vi "Actor Core.vi"(8 "Error In":errorcluster, 11 "CS++RTWatchdogActor in":refnum<class "CS++RTWatchdogActor.lvclass">) -> (0 "Error Out":errorcluster, 3 "Actor out":refnum<class "Actor.lvclass">)   [LabVIEW 2014, in "CS++RTWatchdog.lvlib" / "CS++RTWatchdogActor.lvclass"]
doc: "Periodically resets the watchdog counter to the Watchdog Timeout value. \nStatus changes are send to the caller actor.\n\n(<B>Filename</B>: Actor Framework.lvlib:Actor.lvclass:Actor Core.vi)\n\nReceives messages to the actor, reacts to them, and initiates any error handling that may shut the actor down.\n\nDescendant classes may override this VI to append parallel tasks for the actor to complete while it handles messages. Overrides use the Call Parent Method node."
uses:
  CS++RTWatchdogActor.lvclass
  <vilib>/ActorFramework/Actor/Actor.lvclass
  CS++RTClasses/CS++RTMessageLogger/CS++RTMessageLogger.lvclass
  CS++RTWatchdogActor.lvclass/CS++RTWatchdogActor.ctl
  <vilib>/ActorFramework/Actor/Actor.lvclass/Actor.ctl
  <vilib>/RTwatchdog.llb/Watchdog status enum.ctl
  CS++RTMainActor Messages/Update Watchdog Status Msg/Update Watchdog Status Msg.lvclass/Update Watchdog Status Msg.ctl
  <vilib>/ActorFramework/Message Enqueuer/Message Enqueuer.lvclass/Message Enqueuer.ctl
  <vilib>/ActorFramework/Message Enqueuer/Message Priority.ctl
  <vilib>/ActorFramework/Report Error Msg/Report Error Msg.lvclass/Report Error Msg.ctl
  <vilib>/ActorFramework/Message Enqueuer/Enqueue.vi
  <vilib>/ActorFramework/Message Priority Queue/Priority Enqueue.vi
  <vilib>/ActorFramework/Report Error Msg/Report Error Msg.lvclass
  CS++RTMainActor Messages/Update Watchdog Status Msg/Update Watchdog Status Msg.lvclass
  <vilib>/ActorFramework/Message Enqueuer/Message Enqueuer.lvclass
  CSPP_Core/Classes/CS++BaseClasses/MessageLogger/CS++MessageLogger.lvclass
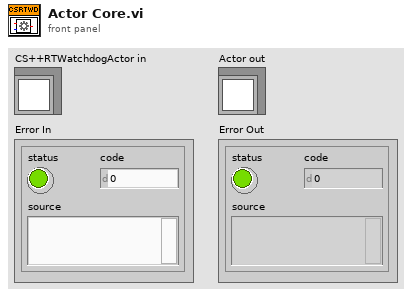
[diagram p1: front panel]
types:
  T1 = typedef "Watchdog expiration actions.ctl" = cluster{"reset":bool, "occurrence":bool, "trigger protocol":enum16{"active high", "active low", "open collector"}, "trigger line":enum16{"none", "line 0", "line 1", "line 2", "line 3", "line 4", "line 5", "line 6", "line 7", "SMB line 0"}, "disable watchdog on VI exit":bool}
  T2 = typedef "Watchdog status enum.ctl" = enum16{"disabled", "expired", "running"}
  T3 = typedef "Actor Framework.lvlib/Message Enqueuer.lvclass/Message Priority.ctl" = enum16{"Low", "Normal", "High"}
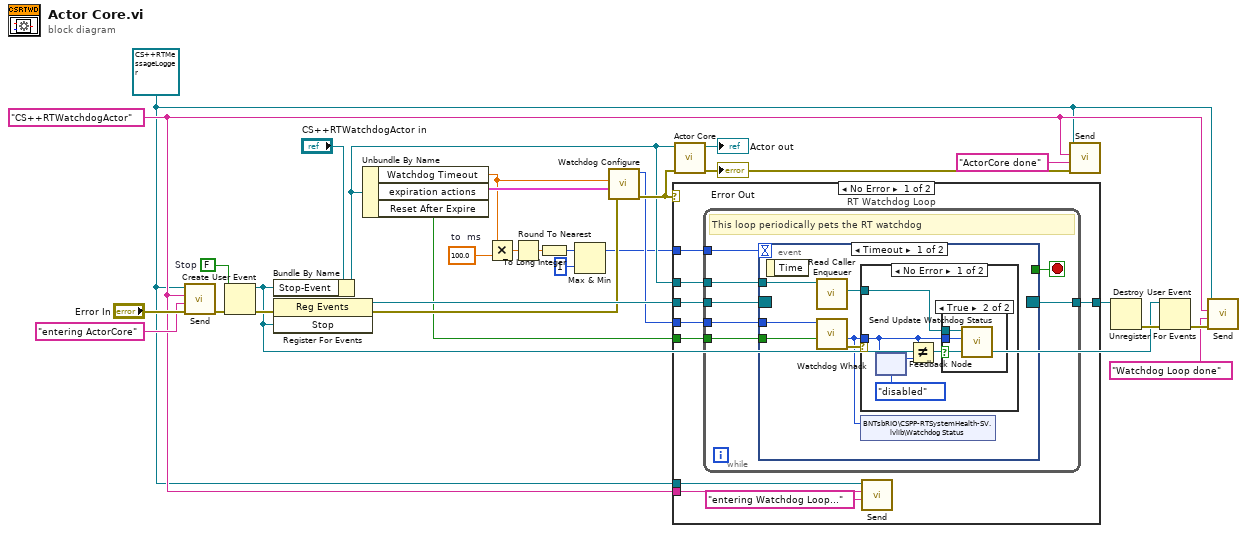
[diagram p0: block diagram]
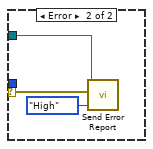
[diagram p3: hidden frame]
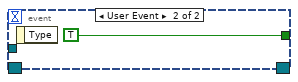
[diagram p4: hidden frame]
diagram:
  w2 = "CS++RTWatchdogActor" ("String to write")
  w1 = refnum<class "CS++RTMessageLogger.lvclass"> refnum ("CS++RTMessageLogger in")
  w15 = 100.0  # to  ms
  w30 = FALSE  # Stop
  n1 = call "Send.vi"("Error In"="Error In", "Message Content"="entering ActorCore" ("String to write"), "Message Tag"=w2, "CS++MessageLogger in"=w1) -> ("Error Out"=w7:errorcluster)  [unwired: 6 in, 1 out]
  n2 = Create User Event(user event datatype=w30, error in=w7) -> (user event=w25:refnum<user-event>, error out=w29:errorcluster)
  n3 = Bundle By Name(cluster="CS++RTWatchdogActor in", "Stop-Event"=w25) -> (w19:refnum<class "CS++RTWatchdogActor.lvclass">)
  n4 = register-events(error in=w29, w25) -> (reference out=w28:refnum<event-registration>, error out=w23:errorcluster)  [unwired: 1 in]
  n5 = Unbundle By Name(w19) -> ("Watchdog Timeout"=w16:dbl, "expiration actions"=w20:T1, "Reset After Expire"=w18:bool)
  n6 = Multiply(x=w16, y=w15) -> (x*y=w14:dbl)
  n7 = Round To Nearest(number=w14) -> (nearest integer value=w11:dbl)
  n8 = To Long Integer(number=w11) -> (32bit integer=w10:i32)
  n9 = Max & Min(x=w10, y=1) -> (max(x,y)=w12:i32)  [unwired: 1 out]
  n10 = call <vilib>:"Watchdog Configure.vi"("error in (no error)"=w23, "expiration actions"=w20, "timeout (1 sec)"=w16) -> ("error out"=w22:errorcluster, "watchdogID"=w21:u64)  [unwired: 1 in, 2 out]
  n11 = case shown="No Error" w22 {
    tunnel: w28 -> [w39 w64]
    tunnel: [w38 w64] -> w27
    tunnel: w21 -> [w37 _]
    tunnel: w19 -> [w36 _]
    tunnel: w18 -> [w35 _]
    tunnel: w12 -> [w34 _]
    tunnel: w2 -> [w32 _]
    tunnel: w1 -> [w31 _]
    frame No Error {
      n12 = while "RT Watchdog Loop" {
        tunnel: w39 -> [w46]
        tunnel: [w45] -> w38
        tunnel: w37 -> [w43]
        tunnel: w36 -> [w42]
        tunnel: w35 -> [w41]
        tunnel: w34 -> [w40]
        stop <- w44 stop-if-true
        # "This loop periodically pets the RT watchdog"
        n13 = event shown="[0] Timeout" {
          selector: w46 -> [_ _]
          dyn-events: [_ _] -> w45
          timeout: w40 -> [_ _]
          tunnel: [_ TRUE] -> w44
          tunnel: w43 -> [w52 _]
          tunnel: w42 -> [w50 _]
          tunnel: w41 -> [w48 _]
          event Timeout {
            n14 = event-data() -> ()  [unwired: 1 in, 1 out]
            n15 = call <vilib>:"Read Caller Enqueuer.vi"("Actor"=w50) -> ("Caller Enqueuer"=w49:refnum<class "Message Enqueuer.lvclass">)  [unwired: 10 in]
            n16 = call <vilib>:"Watchdog Whack.vi"("reset watchdog after expire? (F)"=w48, "watchdogID in"=w52) -> ("error out"=w51:errorcluster, "watchdog status"=w47:T2)  [unwired: 3 in, 1 out]
            n17 = case shown="No Error" w51 {
              selector: w51 -> [_ w62]
              tunnel: w49 -> [w57 w61]
              tunnel: w47 -> [w56 _]
              frame No Error {
                n18 = feedback-in #1(w56) -> ()
                n19 = feedback #1(Watchdog_status_enum."disabled" ("watchdog status")) -> (w55:T2)
                n20 = Not Equal?(x=w56, y=w55) -> (x != y?=w54:bool)
                n21 = case shown="True" w54 {
                  tunnel: w57 -> [_ w59]
                  tunnel: w56 -> [_ w58]
                  frame False {
                  }
                  frame True {
                    n22 = call "Send Update Watchdog Status.vi"("Watchdog Status"=w58, "Message Enqueuer"=w59) -> ()  [unwired: 8 in, 2 out]
                  }
                }
              }
              frame Error {
                n23 = call <vilib>:"Send Error Report.vi"("Message Priority (Normal)"=Message_Priority."High", "Error From Sender"=w62, "Message Enqueuer"=w61) -> ()  [unwired: 8 in, 1 out]
              }
            }
            n24 = shared-variable "BNTsbRIO\\CSPP-RTSystemHealth-SV.lvlib\\Watchdog Status"(w47) -> ()  [unwired: 1 in, 1 out]
          }
          event User Event {
            n25 = event-data() -> ()  [unwired: 1 in, 1 out]
          }
        }
      }
      n26 = call "Send.vi"("Message Content"="entering Watchdog Loop..." ("String to write"), "Message Tag"=w32, "CS++MessageLogger in"=w31) -> ()  [unwired: 7 in, 2 out]
    }
    frame Error {
    }
  }
  n27 = call-parent "Actor Core.vi"("error in"=w22, "Actor in"=w19) -> ("error out"=w3:errorcluster, "Actor out"=→"Actor out":refnum<class "Actor.lvclass">)  [unwired: 8 in]
  "Error Out" <- w3
  n28 = call "Send.vi"("Error In"=w3, "Message Content"="ActorCore done" ("String to write"), "Message Tag"=w2, "CS++MessageLogger in"=w1) -> ()  [unwired: 6 in, 2 out]
  n29 = Unregister For Events(event registration refnum=w27) -> (error out=w26:errorcluster)  [unwired: 1 in]
  n30 = Destroy User Event(user event=w25, error in=w26) -> (error out=w5:errorcluster)
  n31 = call "Send.vi"("Error In"=w5, "Message Content"="Watchdog Loop done" ("String to write"), "Message Tag"=w2, "CS++MessageLogger in"=w1) -> ()  [unwired: 6 in, 2 out]
